vi "InterpretKBCommand.vi"(0 "M2 Increasing":string(combo)="32", 1 "M2 Decreasing":string(combo)="28", 2 "M1 Increasing":string(combo)="13", 3 "M1 Decreasing":string(combo)="10", 4 "M3 Increasing":string(combo)="29", 5 "M3 Decreasing":string(combo)="28", 7 "Key\nValue":i32, 9 "MoveMap":string(combo)="10", 11 "HaltMap":string(combo)="10") -> (6 "M1 Decreasing (#)":i32, 12 "Cluster of Input #s":cluster{i32, i32, i32, i32, i32, i32}, 13 "number":u32, 14 "M2 Increasing (#)":i32, 15 "M1 Increasing (#)":i32, 16 "Move":bool, 17 "Halt":bool, 18 "M2 Decreasing (#)":i32, 19 "Dir Indicator":u32)   [LabVIEW 2020]
panel:
  out "M3 Decreasing (#)":i32
  out "M3 Increasing (#)":i32
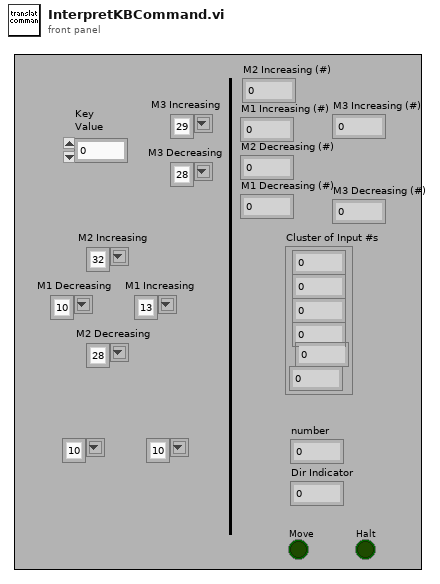
[diagram p1: front panel]
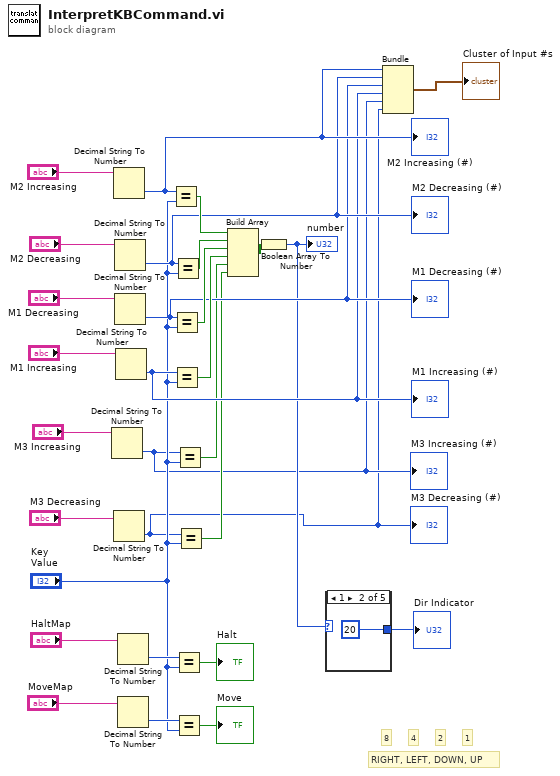
[diagram p0: block diagram]
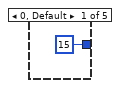
[diagram p2: hidden frame]
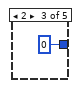
[diagram p3: hidden frame]
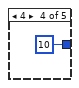
[diagram p4: hidden frame]
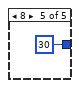
[diagram p5: hidden frame]
diagram:
  # "8"
  # "4"
  # "2"
  # "1"
  # "RIGHT, LEFT, DOWN, UP"
  n1 = Decimal String To Number(string="M3 Increasing") -> (number=w2:i32)  [unwired: 3 out]
  "M3 Increasing (#)" <- w2
  n2 = Decimal String To Number(string="M2 Increasing") -> (number=w20:i32)  [unwired: 3 out]
  "M2 Increasing (#)" <- w20
  n3 = Decimal String To Number(string="M3 Decreasing") -> (number=w1:i32)  [unwired: 3 out]
  "M3 Decreasing (#)" <- w1
  n4 = Decimal String To Number(string="M2 Decreasing") -> (number=w19:i32)  [unwired: 3 out]
  "M2 Decreasing (#)" <- w19
  n5 = Decimal String To Number(string="M1 Decreasing") -> (number=w18:i32)  [unwired: 3 out]
  "M1 Decreasing (#)" <- w18
  n6 = Decimal String To Number(string="M1 Increasing") -> (number=w17:i32)  [unwired: 3 out]
  "M1 Increasing (#)" <- w17
  n7 = Decimal String To Number(string="HaltMap") -> (number=w13:i32)  [unwired: 3 out]
  n8 = Decimal String To Number(string="MoveMap") -> (number=w11:i32)  [unwired: 3 out]
  n9 = Equal?(x=w20, y="Key\nValue") -> (x = y?=w25:bool)
  n10 = Equal?(x=w18, y="Key\nValue") -> (x = y?=w23:bool)
  n11 = Equal?(x=w17, y="Key\nValue") -> (x = y?=w22:bool)
  n12 = Equal?(x=w19, y="Key\nValue") -> (x = y?=w24:bool)
  n13 = Equal?(x=w13, y="Key\nValue") -> (x = y?=→"Halt":bool)
  n14 = Equal?(x=w11, y="Key\nValue") -> (x = y?=→"Move":bool)
  n15 = Equal?(x=w2, y="Key\nValue") -> (x = y?=w6:bool)
  n16 = Equal?(x=w1, y="Key\nValue") -> (x = y?=w3:bool)
  n17 = Build Array(w25, w24, w23, w22, w6, w3) -> (w21:bool[])
  n18 = Boolean Array To Number(Boolean array=w21) -> (number=w15:u32)
  "number" <- w15
  n19 = case shown="1" w15 {
    tunnel: [u32 15 ("number") u32 20 ("number") u32 0 ("number") u32 10 ("number") u32 30 ("number")] -> w14
    frame 0, Default {
    }
    frame 1 {
    }
    frame 2 {
    }
    frame 4 {
    }
    frame 8 {
    }
  }
  "Dir Indicator" <- w14
  n20 = Bundle(w20, w19, w18, w17, w2, w1) -> (→"Cluster of Input #s":cluster{i32, i32, i32, i32, i32, i32})  [unwired: 1 out]
